vi "Async Update & Write.vi"(1 "Minor Frame Freq":u16 caption="Minor Frame Time", 6 "Continuous Tx":bool, 8 "error in":errorcluster, 9 "Interupt Q":refnum<queue>, 10 "Frame Info Array":T1[](array[typedef]), 11 "Visa":refnum<visa-resource-name>) -> (0 "error out":errorcluster, 2 "Frame Info Array":T1[](array[typedef]), 3 "Stop":bool)   [LabVIEW 2024]
doc: "All Rights Reserved © 2017 SyncSols"
uses:
  Controls/Async Frame Info Cluster.ctl
  Controls/Async Message Info Cluster.ctl
  TCP Engine/Controls/TCP Engine Serial Interupt Cluster.ctl
  TCP Engine/TCP Engine.lvlib
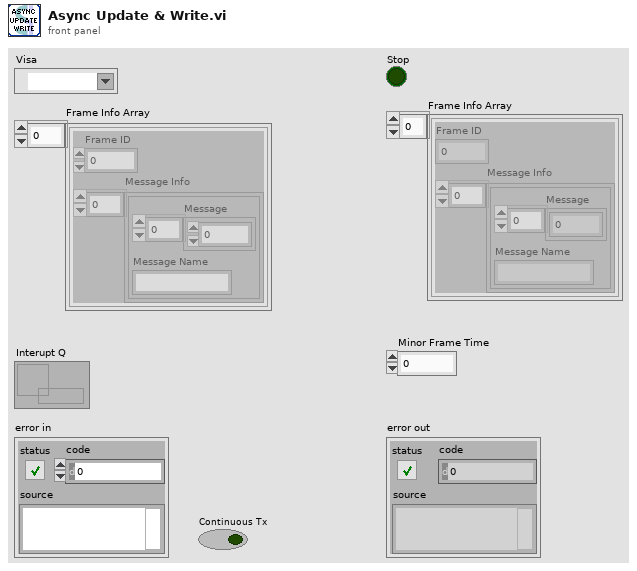
[diagram p1: front panel]
types:
  T1 = typedef "Async Frame Info Cluster.ctl" = cluster{"Frame ID":u16, "Message Info":T2[]}
  T2 = typedef "Async Message Info Cluster.ctl" = cluster{"Message":u8[], "Message Name":string}
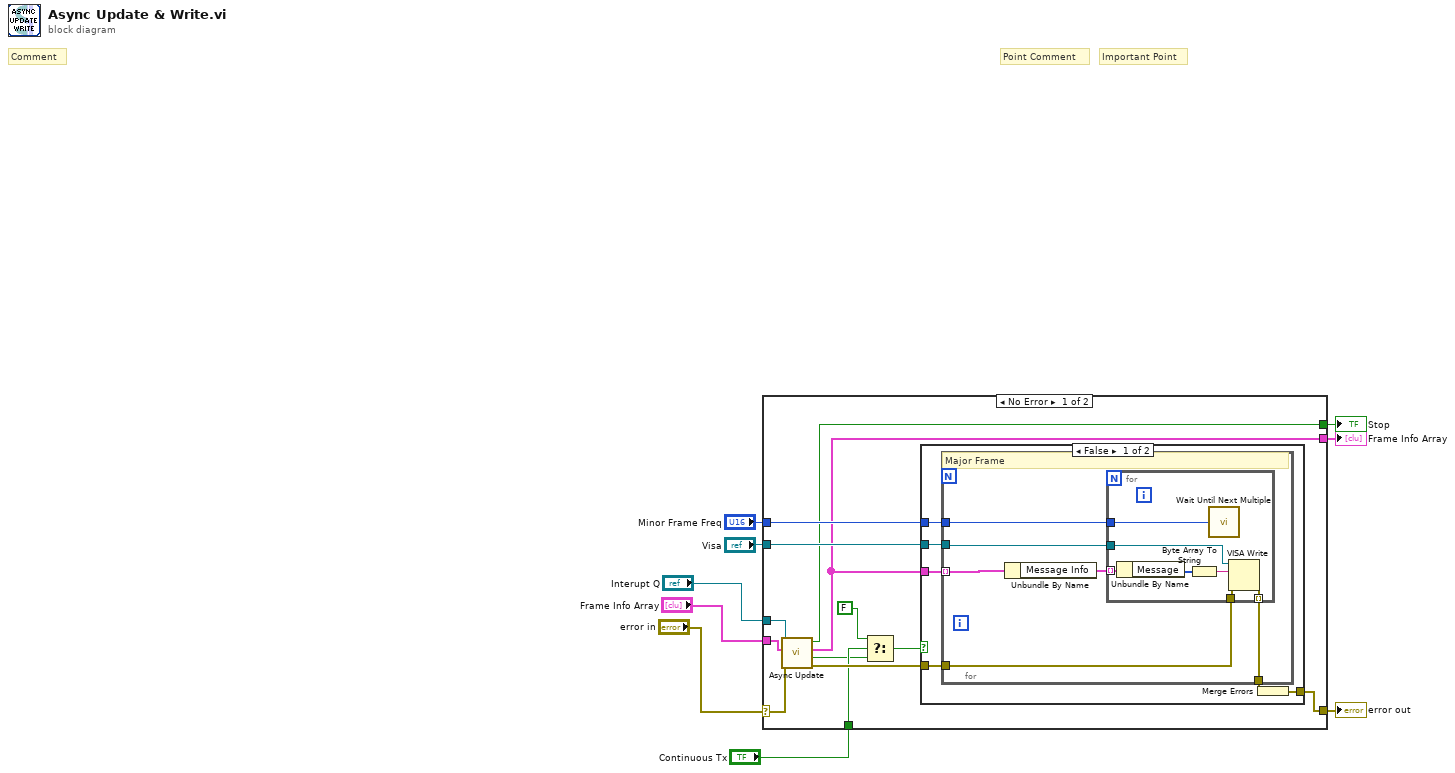
[diagram p0: block diagram]
diagram:
  # "Important Point"
  # "Point Comment"
  # "Comment"
  n1 = case shown="No Error" "error in" {
    selector: "error in" -> [w19 w44]
    tunnel: [w14 w44] -> w6
    tunnel: "Visa" -> [w22 _]
    tunnel: "Minor Frame Freq" -> [w21 _]
    tunnel: [w15 w43] -> w5
    tunnel: [w16 _] -> w4
    tunnel: "Frame Info Array" -> [w20 w43]
    tunnel: "Interupt Q" -> [w18 _]
    tunnel: "Continuous Tx" -> [w13 _]
    frame No Error {
      n2 = call "Async Update.vi"("error in"=w19, "Frame Info Array"=w20, "Interupt Q"=w18) -> ("error out"=w17:errorcluster, "timed out?"=w10:bool, "Frame Info Array"=w15:T1[], "Stop"=w16:bool)  [unwired: 5 in]
      n3 = Select(t=FALSE ("Continuous Tx"), s=w13, f=w10) -> (s? t:f=w11:bool)
      n4 = case shown="False" w11 {
        tunnel: w22 -> [w28 _]
        tunnel: w21 -> [w27 _]
        tunnel: w17 -> [w26 w42]
        tunnel: w15 -> [w25 _]
        tunnel: [w23 w42] -> w14
        frame False {
          n5 = for {
            tunnel: w28 -> [w33]
            tunnel: w27 -> [w29]
            tunnel: [w32] -> w24
            tunnel: w25 -> [w30] mode=indexing
            tunnel: w26 -> [w31]
            # "Major Frame"
            n6 = Unbundle By Name(w30) -> ("Message Info"=w34:T2[])
            n7 = for {
              tunnel: w34 -> [w41] mode=indexing
              tunnel: w33 -> [w38]
              tunnel: [w37] -> w32 mode=indexing
              tunnel: w31 -> [w36]
              tunnel: w29 -> [w35]
              n8 = Unbundle By Name(w41) -> ("Message"=w40:u8[])
              n9 = Byte Array To String(unsigned byte array=w40) -> (string=w39:string)
              n10 = call "Wait Until Next Multiple"("Count(mSec)"=w35) -> ()  [unwired: 1 out]
              n11 = VISA Write(VISA resource name=w38, write buffer=w39, error in (no error)=w36) -> (error out=w37:errorcluster)  [unwired: 2 out]
            }
          }
          n12 = Merge Errors(w24) -> (w23:errorcluster)
        }
        frame True {
        }
      }
    }
    frame Error {
    }
  }
  "error out" <- w6
  "Stop" <- w4
  "Frame Info Array" <- w5
